vi "Music Library To Artist Library Display.vi"(8 "error in (no error)":errorcluster, 11 "Artist Library":refnum<class "MusicElementLibrary.lvclass">) -> (0 "error out":errorcluster, 3 "Music Library Display Array":T1[](array[typedef]) {"Duration (s)" format="%<%M:%S>T"})   [LabVIEW 2015, in "SongBrowserActor.lvlib" / "SongBrowserActor.lvclass"]
uses:
  SongBrowserActor.lvclass
  controls/Music Library Element Display.ctl
  file/MusicElement/Song/Song Duration.ctl
  file/MusicElement/MusicElementLibrary/MusicElementLibrary.lvclass
  file/MusicElement/MusicElementLibrary/MusicElementLibrary.lvclass/MusicElementLibrary.ctl
  file/MusicElement/MusicElementLibrary/SongLibrary/SongLibrary.lvclass
  file/MusicElement/MusicElement.lvclass/MusicElement.ctl
  file/MusicElement/MusicElementLibrary/Read Music Element Library.vi
  file/MusicElement/MusicElement.lvclass
  file/MusicElement/Song/Song.lvclass
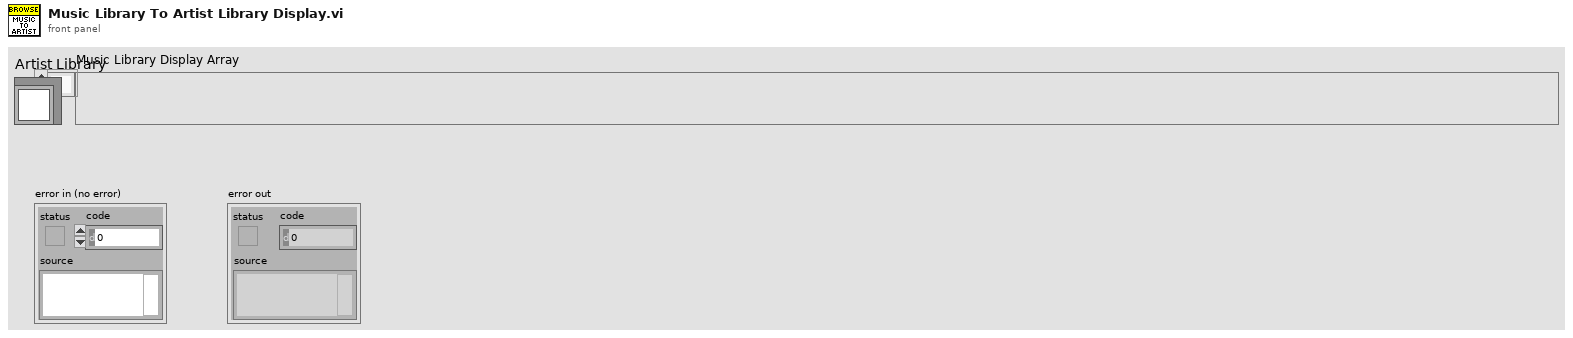
[diagram p1: front panel]
types:
  T1 = typedef "Music Library Element Display.ctl" = cluster{"Name":string, "Details":string, "Duration (s)":T2, "Click":bool}
  T2 = typedef "Song.lvclass/Song Duration.ctl" = timestamp
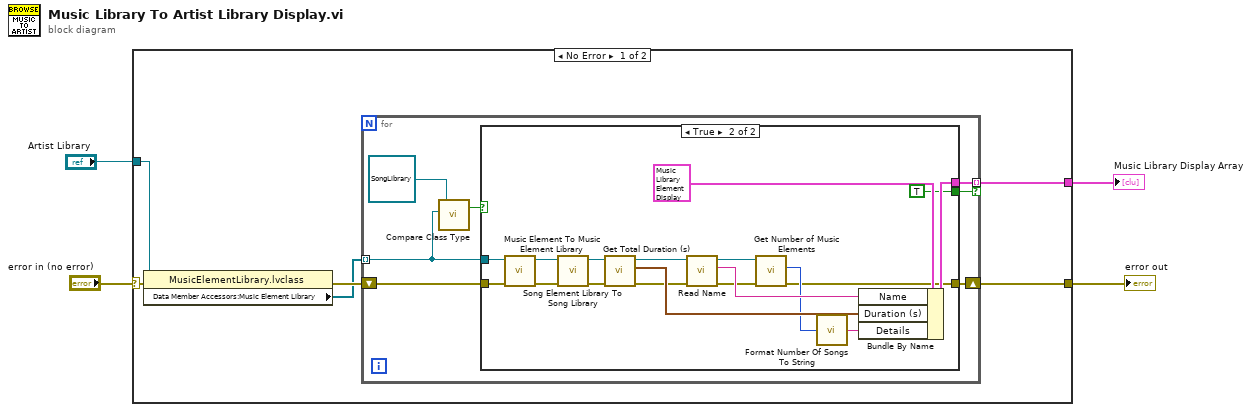
[diagram p0: block diagram]
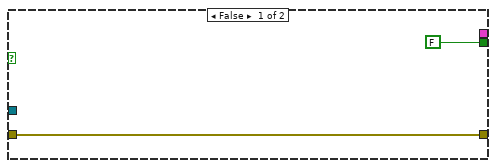
[diagram p2: hidden frame]
diagram:
  n1 = case shown="No Error" "error in (no error)" {
    selector: "error in (no error)" -> [w10 w38]
    tunnel: [w8 w38] -> w3
    tunnel: "Artist Library" -> [w9 _]
    tunnel: [w7 _] -> w2
    frame No Error {
      n2 = property class="MusicElementLibrary.lvclass"(reference=w9, error in=w10) -> (error out=w6:errorcluster, "Data Member Accessors:Music Element Library"=w5:refnum<class "MusicElement.lvclass">[])  [unwired: 1 out]
      n3 = for {
        shift-right: [w15] -> w8
        shift-left: w6 -> [w16]
        tunnel: [w17] -> w7 mode=indexing if=w11
        tunnel: w5 -> [w12] mode=indexing
        n4 = call "Compare Class Type.vi"("MusicElement Check"=w12, "MusicElement in"=refnum<class "SongLibrary.lvclass"> refnum ("SongLibrary out")) -> ("Same Class Type?"=w14:bool)  [unwired: 3 in]
        n5 = case shown="True" w14 {
          tunnel: [_ w37] -> w17
          tunnel: w16 -> [w18 w33]
          tunnel: w12 -> [_ w32]
          tunnel: [w18 w21] -> w15
          tunnel: [FALSE TRUE] -> w11
          frame False {
          }
          frame True {
            n6 = call "Music Element To Music Element Library.vi"("error in (no error)"=w33, "MusicElement"=w32) -> ("error out"=w31:errorcluster, "MusicElementLibrary out"=w30:refnum<class "MusicElementLibrary.lvclass">)  [unwired: 8 in]
            n7 = call "Song Element Library To Song Library.vi"("error in (no error)"=w31, "MusicElementLibrary"=w30) -> ("error out"=w29:errorcluster, "SongLibrary out"=w28:refnum<class "SongLibrary.lvclass">)  [unwired: 8 in]
            n8 = call "Get Total Duration (s).vi"("error in (no error)"=w29, "SongLibrary in"=w28) -> ("error out"=w27:errorcluster, "Duration (s)"=w35:T2, "SongLibrary out"=w26:refnum<class "SongLibrary.lvclass">)  [unwired: 7 in]
            n9 = call "Read Name.vi"("error in (no error)"=w27, "MusicElement in"=w26) -> ("error out"=w24:errorcluster, "Name"=w25:string, "MusicElement out"=w23:refnum<class "SongLibrary.lvclass">)  [unwired: 7 in]
            n10 = call "Get Number of Music Elements.vi"("error in (no error)"=w24, "MusicElementLibrary in"=w23) -> ("error out"=w21:errorcluster, "Size"=w22:i32)  [unwired: 7 in, 1 out]
            n11 = call "Format Number Of Songs To String.vi"("Number Of Songs"=w22) -> ("Formatted"=w34:string)
            n12 = Bundle By Name(cluster=T1 {"Name"="", "Details"="", "Duration (s)"=timestamp(0 s since 1904-01-01), "Click"=FALSE} ("Element"), "Name"=w25, "Duration (s)"=w35, "Details"=w34) -> (w37:T1)
          }
        }
      }
    }
    frame Error {
    }
  }
  "error out" <- w3
  "Music Library Display Array" <- w2
